vi "Feature Extractor.vi"() -> ()   [LabVIEW 2020]
uses:
  <vilib>/Utility/file.llb/Write Delimited Spreadsheet (string).vi
  <vilib>/Utility/file.llb/Read Delimited Spreadsheet (string).vi
panel:
  in  "Tab Control":enum32{"Measurements", "Settings"}(tab)
  in  "Feature checkmarks":cluster{"Boolean":bool, "String":string}[](array[cluster])=[{"Boolean"=FALSE, "String"="monkey (other animal)"}, {"Boolean"=FALSE, "String"="face (non-face)"}, {"Boolean"=FALSE, "String"="baby (adult)"}]
  in  "next":bool
  in  "previous":bool
  in  "Picture":i32
  out "number of pictures":i32=5
  in  "add object":bool
  in  "save all":bool
  in  "delete object":bool
  in  "next object":bool
  in  "previous object":bool
  in  "Object":i32
  in  "Category":u16(ring) items=["grooming", "aggression", "monkey_play", "group", "mating", "baby_monkey", "animals_playing", "hiding"]
  in  "Save Settings":bool
  in  "Pictures folder path":path=path "C:/Users/Azat/Documents/Monkey Research/Face Grabber/Example"
  in  "Features file path":path=path "C:/Users/Azat/Documents/Monkey Research/Face Grabber/Example/metrics.csv"
  in  "Categories file path":path=path "C:/Users/Azat/Documents/Monkey Research/Face Grabber/Example/stimuli categories.csv"
  in  "show in folder":bool
  in  "new table":bool
  in  "open table":bool
  out "Categories":string[](array[string])=["grooming", "aggression", "monkey_play", "group", "mating", "baby_monkey", "animals_playing", "hiding"]
  out "All Files in Dir":path[](array[path])=[path "C:/Users/Azat/Documents/Monkey Research/Face Grabber/Example/001_monkey_grooming.jpg", path "C:/Users/Azat/Documents/Monkey Research/Face Grabber/Example/017_monkey_aggression.jpg", path "C:/Users/Azat/Documents/Monkey Research/Face Grabber/Example/033_monkey_playing.jpg", path "C:/Users/Azat/Documents/Monkey Research/Face Grabber/Example/049_monkey_group.jpg", path "C:/Users/Azat/Documents/Monkey Research/Face Grabber/Example/089_baby_monkey.jpg"]
  out "Results table":string[][](table)
  in  "Results table file path":path=path "C:/Users/Azat/Documents/Monkey Research/Face Grabber/Example/results.csv"
  out "contours":T1(array[cluster])
  in  "stop":bool
  out "Image":T2(plugin-control)
  # "/"
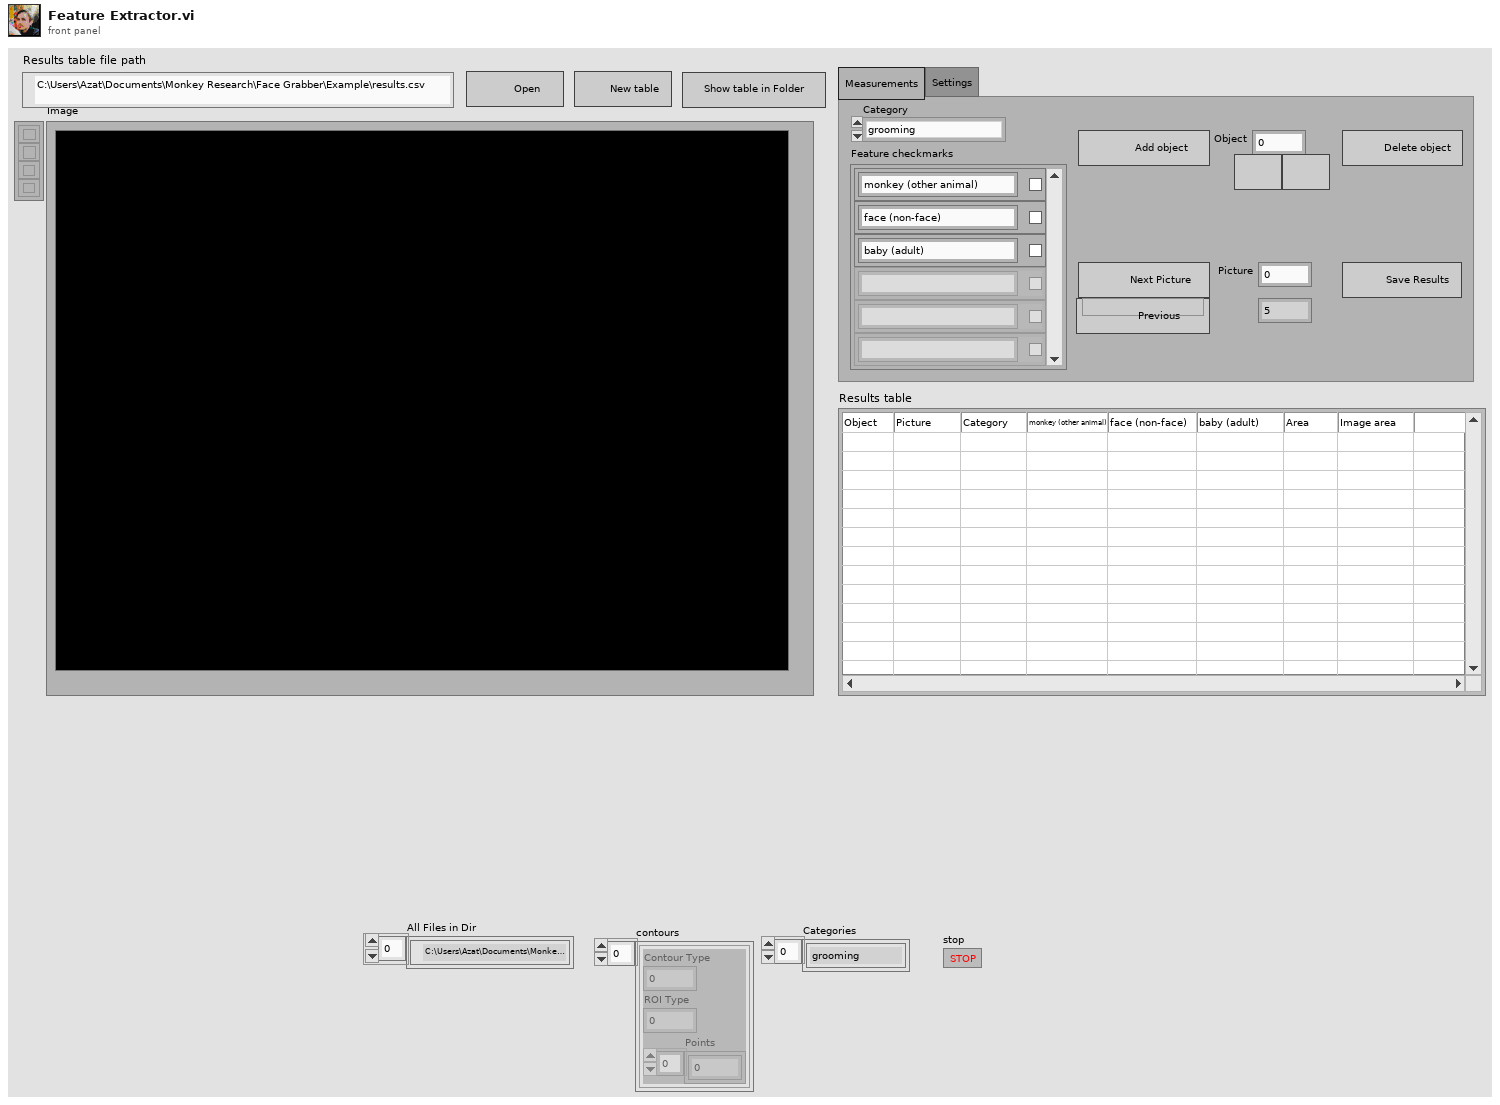
[diagram p1: front panel]
types:
  T1 = cluster{"Contour Type":u32, "ROI Type":u32, "Points":i32[]}[]
  T2 = typedef "IMAQ Image.ctl" = refnum<image>
  T3 = cluster{"Global Rectangle":i32[], "Contours":cluster{"Contour Type":u32, "ROI Type":u32, "Points":i32[]}[]}
  T4 = cluster{"Pictures":path, "results table":path, "Metrics":path, "Categories":path}
  T5 = cluster{"appended path":path, "appended path":path, "appended path":path, "appended path":path}
  T6 = cluster{"[0]":path, "[1]":path, "[2]":path, "[3]":path, "[4]":path, "[5]":path, "[6]":path, "[7]":path, "[8]":path}
  T7 = cluster{"Global Rectangle":i32[], cluster{"Contour Type":u32, "ROI Type":u32, "Points":i32[]}[]}
  T8 = cluster{"Contour Type":u32, "ROI Type":u32, "Points":i32[]}
  T9 = cluster{"Pictures folder path":path, "selected path":path, "Features file path":path, "Categories file path":path}
  T10 = cluster{"Pictures folder path":path, "Results table file path":path, "Features file path":path, "Categories file path":path}
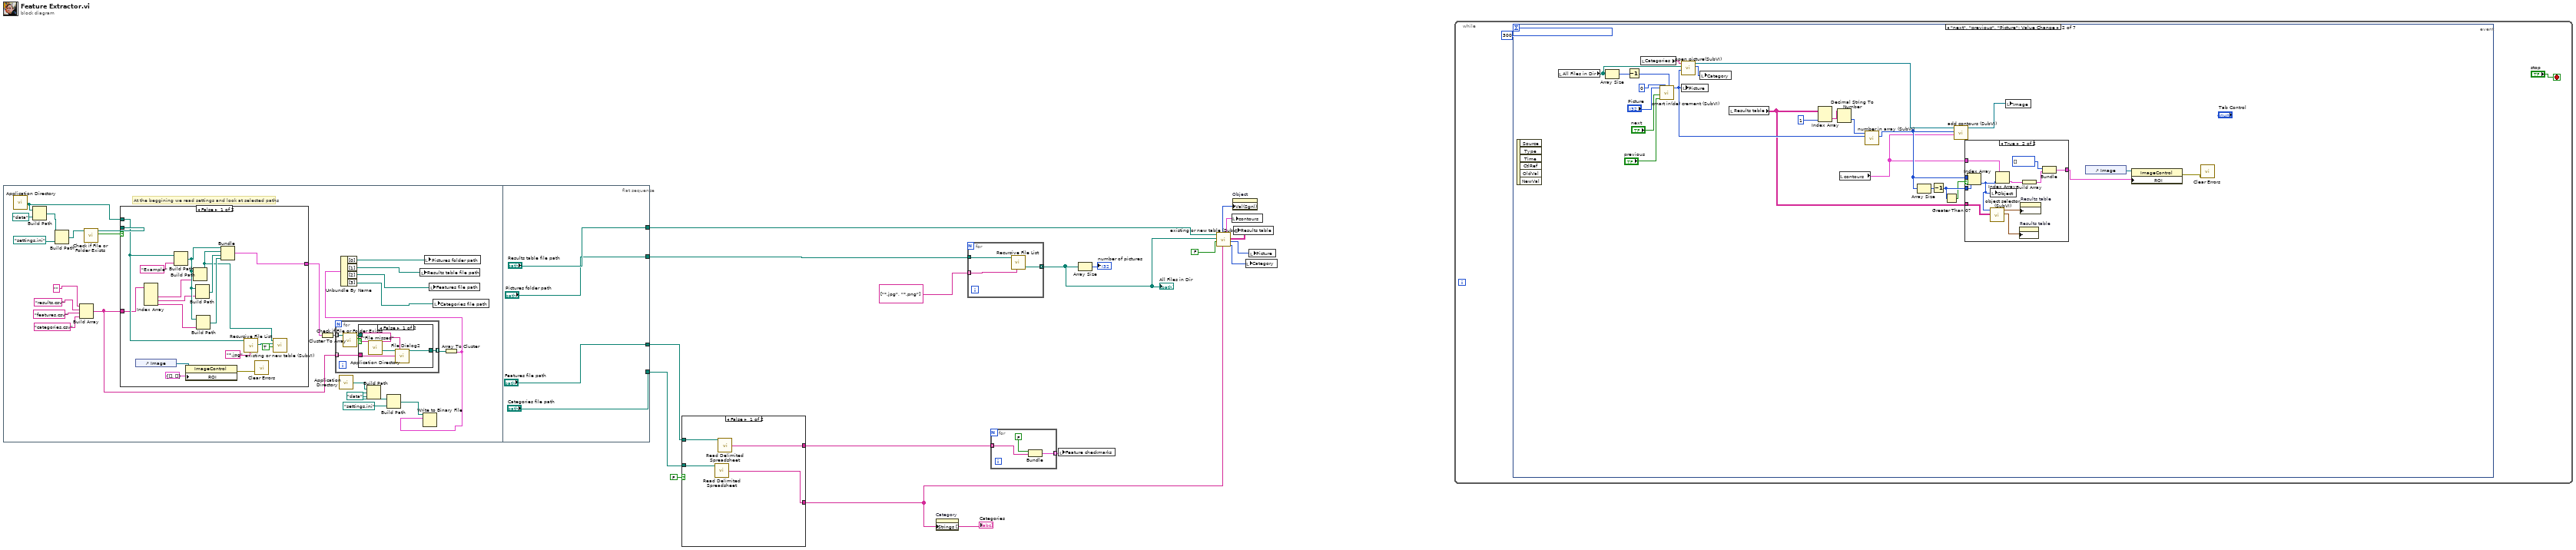
[diagram p0: block diagram]
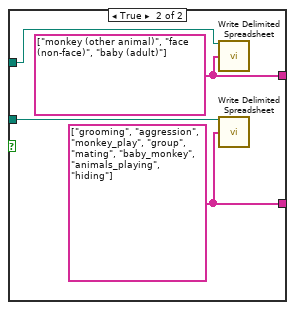
[diagram p2: hidden frame]
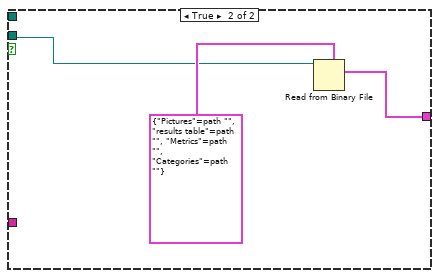
[diagram p4: hidden frame]
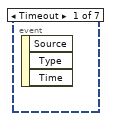
[diagram p5: hidden frame]
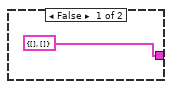
[diagram p6: hidden frame]
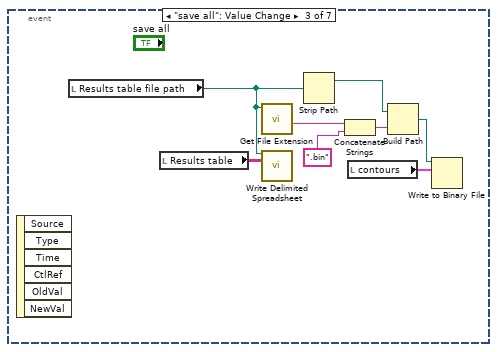
[diagram p7: hidden frame]
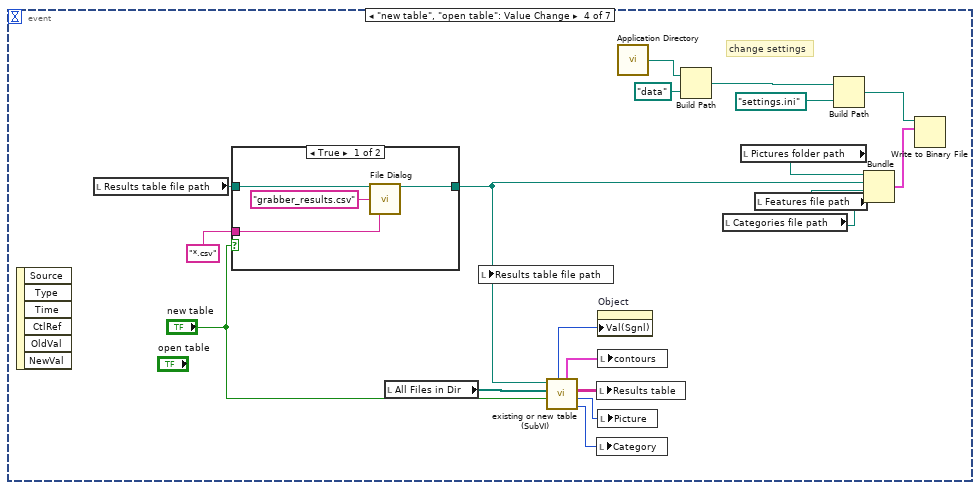
[diagram p8: hidden frame]
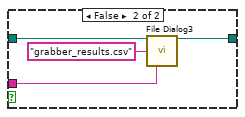
[diagram p9: hidden frame]
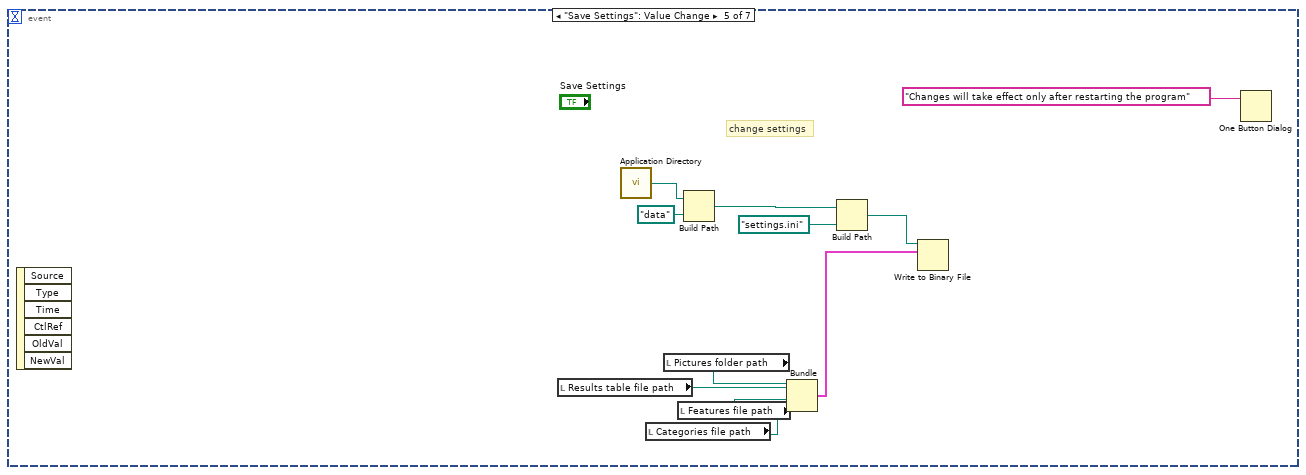
[diagram p10: hidden frame]
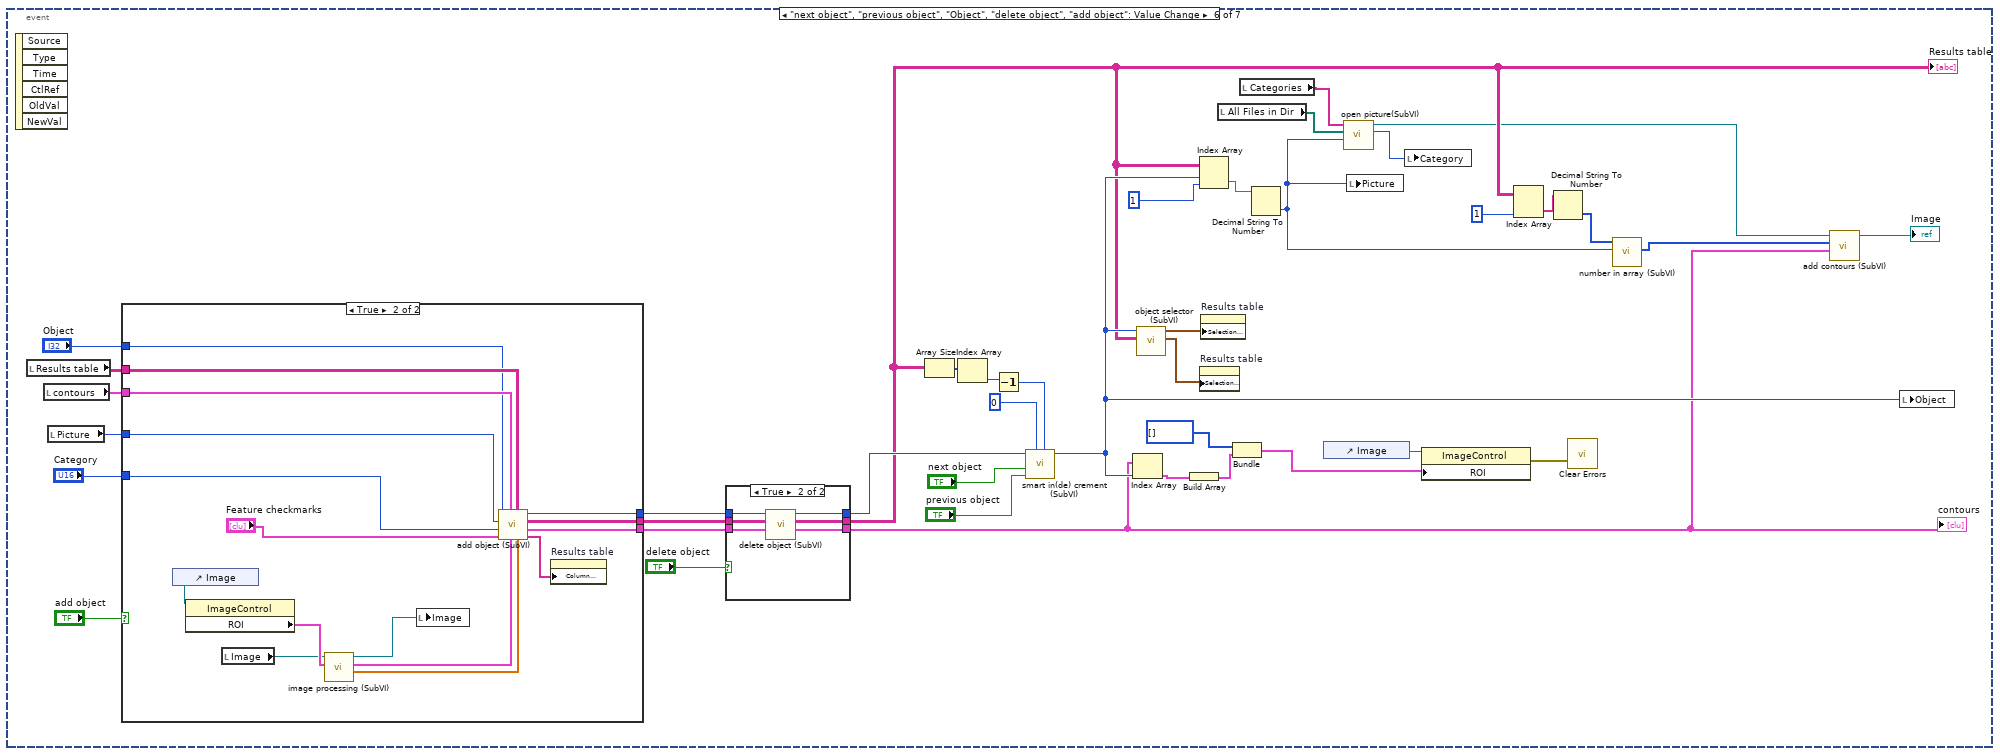
[diagram p11: hidden frame]
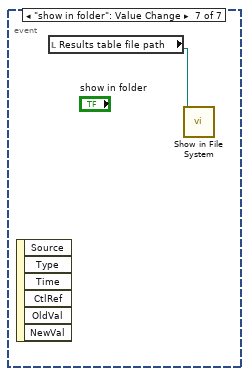
[diagram p14: hidden frame]
diagram:
  n1 = flat-sequence {
    tunnel: ["Results table file path"] -> w11
    tunnel: ["Pictures folder path"] -> w10
    tunnel: ["Features file path"] -> w3
    tunnel: ["Categories file path"] -> w2
    frame #0 {
      # "At the beggining we read settings and look at selected paths"
      n2 = call <vilib>:"Application Directory.vi"() -> ("Application Directory"=w32:path)
      n3 = Build Path(base path=w32, name or relative path=path "data") -> (appended path=w35:path)
      n4 = Build Path(base path=w35, name or relative path=path "settings.ini") -> (appended path=w38:path)
      n5 = Build Array("" ("default name"), "results.csv" ("default name"), "features.csv" ("default name"), "categories.csv" ("default name")) -> (w25:string[])
      n6 = call <vilib>:"Check if File or Folder Exists.vi"("path"=w38) -> ("file or folder exists?"=w39:bool, "dup path"=w40:path)  [unwired: 8 in, 1 out]
      n7 = case shown="False" w39 {
        tunnel: w40 -> [_ w71]
        tunnel: w32 -> [w62 _]
        tunnel: [w69 w70] -> w31
        tunnel: w25 -> [w56 _]
        frame False {
          n8 = control-ref of="Image"() -> (w58:refnum<vi>)
          n9 = Index Array(array=w56) -> (element #2=w55:string, element #3=w54:string, element #4=w53:string)  [unwired: 4 in, 1 out]
          n10 = Build Path(base path=w62, name or relative path="Example" ("default name")) -> (appended path=w65:path)
          n11 = property class="ImageControl"(reference=w58, "ROI"=T3 {"Global Rectangle"=[], "Contours"=[]}) -> (error out=w59:errorcluster)  [unwired: 1 in, 1 out]
          n12 = Build Path(base path=w65, name or relative path=w55) -> (appended path=w60:path)
          n13 = Build Path(base path=w65, name or relative path=w54) -> (appended path=w67:path)
          n14 = Build Path(base path=w65, name or relative path=w53) -> (appended path=w66:path)
          n15 = Bundle("appended path"=w65, "appended path"=w60, "appended path"=w67, "appended path"=w66) -> (w69:T5)  [unwired: 1 in]
          n16 = call <vilib>:"Recursive File List.vi"("pattern"="*.jpg", "Folder Path"=w62) -> ("All Files in Dir"=w63:path[])  [unwired: 5 in, 4 out]
          n17 = call <vilib>:"Clear Errors.vi"("error in (no error)"=w59) -> ()  [unwired: 5 in, 2 out]
          n18 = call "existing or new table (SubVI).vi"("new table?"=TRUE, "All Files in Dir (in)"=w63, "table"=w60) -> ()  [unwired: 4 in, 5 out]
        }
        frame True {
          n19 = Read from Binary File(5:T4 {"Pictures"=path "", "results table"=path "", "Metrics"=path "", "Categories"=path ""} ("output cluster"), 11:w71) -> (2:w70:T4)  [unwired: 4 in, 3 out]
        }
      }
      n20 = Cluster To Array(cluster=w31) -> (array=w30:path[])
      n21 = for {
        tunnel: w30 -> [w47] mode=indexing
        tunnel: w25 -> [w45] mode=indexing
        tunnel: [w43] -> w24 mode=indexing
        n22 = call <vilib>:"Check if File or Folder Exists.vi"("path"=w47) -> ("file or folder exists?"=w46:bool, "dup path"=w44:path)  [unwired: 8 in, 1 out]
        n23 = case shown="False" w46 {
          tunnel: w45 -> [w51 _]
          tunnel: [w48 w52] -> w43
          tunnel: w44 -> [_ w52]
          frame False {
            n24 = call <vilib>:"Application Directory.vi"() -> ("Application Directory"=w49:path)
            n25 = call "File Dialog2"("start path"=w49, "prompt"="File missed", "default name"=w51) -> ("selected path"=w48:path)  [unwired: 9 in, 3 out]
          }
          frame True {
          }
        }
      }
      n26 = call <vilib>:"Application Directory.vi"() -> ("Application Directory"=w22:path)
      n27 = Build Path(base path=w22, name or relative path=path "data") -> (appended path=w21:path)
      n28 = Build Path(base path=w21, name or relative path=path "settings.ini") -> (appended path=w23:path)
      n29 = Array To Cluster(array=w24) -> (cluster=w18:T6)
      n30 = Unbundle By Name(w18) -> ("[0]"=w41:path, "[1]"=w42:path, "[2]"=w34:path, "[3]"=w33:path)
      n31 = local write "Results table file path"(w42) -> ()
      n32 = Write to Binary File(file (use dialog)=w23, data=w18) -> ()  [unwired: 4 in, 3 out]
      n33 = local write "Pictures folder path"(w41) -> ()
      n34 = local write "Features file path"(w34) -> ()
      n35 = local write "Categories file path"(w33) -> ()
    }
    frame #1 {
    }
  }
  n36 = case shown="False" FALSE {
    tunnel: [w77 w81] -> w9
    tunnel: [w79 w84] -> w7
    tunnel: w2 -> [w80 w83]
    tunnel: w3 -> [w78 w82]
    frame False {
      n37 = call-poly <vilib>:"Read Delimited Spreadsheet.vi"("file path (dialog if empty)"=w80) -> ("first row"=w79:string[])  [unwired: 9 in, 5 out]
      n38 = call-poly <vilib>:"Read Delimited Spreadsheet.vi"("file path (dialog if empty)"=w78) -> ("first row"=w77:string[])  [unwired: 9 in, 5 out]
    }
    frame True {
      w81 = string[] ["monkey (other animal)", "face (non-face)", "baby (adult)"]
      w84 = string[] ["grooming", "aggression", "monkey_play", "group", "mating", "baby_monkey", "animals_playing", "hiding"] ("Strings []")
      n39 = call-poly <vilib>:"Write Delimited Spreadsheet.vi"("file path (dialog if empty)"=w82, "1D data"=w81) -> ()  [unwired: 12 in, 2 out]
      n40 = call-poly <vilib>:"Write Delimited Spreadsheet.vi"("file path (dialog if empty)"=w83, "1D data"=w84) -> ()  [unwired: 12 in, 2 out]
    }
  }
  "Categories" <- w7
  n41 = property on="Category" class="Ring (strict)"("Strings []"=w7) -> ()  [unwired: 2 in, 2 out]
  n42 = for {
    tunnel: [w87] -> w12 mode=concatenating
    tunnel: w10 -> [w86]
    tunnel: string[] ["*.jpg", "*.png"] -> [w85] mode=indexing
    n43 = call <vilib>:"Recursive File List.vi"("pattern"=w85, "Folder Path"=w86) -> ("All Files in Dir"=w87:path[])  [unwired: 5 in, 4 out]
  }
  "All Files in Dir" <- w12
  n44 = for {
    tunnel: w9 -> [w89] mode=indexing
    tunnel: [w88] -> w8 mode=indexing
    n45 = Bundle(FALSE, "String"=w89) -> (w88:cluster{bool, "String":string})  [unwired: 1 in]
  }
  n46 = local write "Feature checkmarks"(w8) -> ()
  n47 = Array Size(array=w12) -> (size(s)=→"number of pictures":i32)
  n48 = call "existing or new table (SubVI).vi"("Categories (in)"=w7, "new table?"=FALSE, "All Files in Dir (in)"=w12, "table"=w11) -> ("category"=w13:i32, "picture"=w5:i32, "text table"=w14:string[][], "contours"=w15:T1, "Object"=w4:i32)  [unwired: 3 in]
  n49 = local write "contours"(w15) -> ()
  n50 = property on="Object" class="DigNum (strict)"("Val(Sgnl)"=w4) -> ()  [unwired: 2 in, 2 out]
  n51 = local write "Results table"(w14) -> ()
  n52 = local write "Category"(w13) -> ()
  n53 = local write "Picture"(w5) -> ()
  n54 = while {
    stop <- "stop" stop-if-true
    n55 = event shown="[1] \"next\", \"previous\", \"Picture\": Value Change" {
      selector: _ -> [_ _ _ _ _ _ _]
      dyn-events: _ -> [_ _ _ _ _ _ _]
      timeout: 300 -> [_ _ _ _ _ _ _]
      event Timeout {
        n56 = event-data() -> ()  [unwired: 1 in, 3 out]
      }
      event "next", "previous", "Picture": Value Change {
        n57 = event-data() -> ()  [unwired: 1 in, 6 out]
        n58 = local read "All Files in Dir"() -> (w113:path[])
        n59 = Array Size(array=w113) -> (size(s)=w114:i32)
        n60 = Decrement(x=w114) -> (x-1=w110:i32)
        n61 = local read "Categories"() -> (w115:string[])
        n62 = call "smart in(de) crement (SubVI).vi"("upper limit in"=w110, "lower limit"=0, "previous object"="previous", "next object"="next", "Object"="Picture") -> ("Object out"=w104:i32)  [unwired: 6 in]
        n63 = call "open picture(SubVI).vi"("Picture number"=w104, "All Files in Dir"=w113, "Categories"=w115) -> ("Category"=w116:i32, "Image"=w102:T2)  [unwired: 7 in]
        n64 = local write "Picture"(w104) -> ()
        n65 = local write "Category"(w116) -> ()
        n66 = local read "Results table"() -> (w93:string[][])
        n67 = Index Array(array=w93, index (col)=1 ("disabled index (col)")) -> (element=w106:string[])  [unwired: 1 in]
        n68 = Decimal String To Number(string=w106) -> (number=w105:i32[])  [unwired: 2 in, 1 out]
        n69 = local read "contours"() -> (w99:T1)
        n70 = call "number in array (SubVI).vi"("Numeric"=w104, "Array"=w105) -> ("indexes"=w101:i32[])  [unwired: 8 in, 1 out]
        n71 = Array Size(array=w101) -> (size(s)=w100:i32)
        n72 = Decrement(x=w100) -> (x-1=w98:i32)
        n73 = Greater Than 0?(x=w98) -> (x > 0?=w94:bool)
        n74 = call "add contours (SubVI).vi"("contours in"=w99, "indexes"=w101, "Refnum in"=w102) -> ("Refnum out"=w103:T2)  [unwired: 8 in]
        n75 = case shown="True" w94 {
          tunnel: w101 -> [_ w128]
          tunnel: w99 -> [_ w127]
          tunnel: w98 -> [_ w119]
          tunnel: [T7 {"Global Rectangle"=[], []} ("output cluster") w126] -> w96
          tunnel: w93 -> [_ w120]
          frame False {
          }
          frame True {
            n76 = Index Array(array=w128, index=w119) -> (element=w118:i32)
            n77 = call "object selector (SubVI).vi"("output array"=w120, "Numeric"=w118) -> ("Cluster"=w122:cluster{"Object":i32, i32}, "Cluster 2"=w121:cluster{i32, "Object":i32})  [unwired: 8 in]
            n78 = local write "Object"(w118) -> ()
            n79 = Index Array(array=w127, index=w118) -> (element=w124:T8)
            n80 = property on="Results table" class="Tbl (strict)"("Selection Size"=w122) -> ()  [unwired: 2 in, 2 out]
            n81 = property on="Results table" class="Tbl (strict)"("Selection Start"=w121) -> ()  [unwired: 2 in, 2 out]
            n82 = Build Array(w124) -> (w125:T1)
            n83 = Bundle("Global Rectangle"=i32[] [], w125) -> (w126:T7)  [unwired: 1 in]
          }
        }
        n84 = local write "Image"(w103) -> ()
        n85 = control-ref of="Image"() -> (w95:refnum<vi>)
        n86 = property class="ImageControl"(reference=w95, "ROI"=w96) -> (error out=w97:errorcluster)  [unwired: 1 in, 1 out]
        n87 = call <vilib>:"Clear Errors.vi"("error in (no error)"=w97) -> ()  [unwired: 5 in, 2 out]
      }
      event "save all": Value Change {
        n88 = event-data() -> ()  [unwired: 1 in, 6 out]
        n89 = local read "Results table file path"() -> (w129:path)
        n90 = local read "Results table"() -> (w130:string[][])
        n91 = call <vilib>:"Get File Extension.vi"("file"=w129) -> ("filename without extension"=w135:string)  [unwired: 6 in, 4 out]
        n92 = call-poly <vilib>:"Write Delimited Spreadsheet.vi"("file path (dialog if empty)"=w129, "2D data"=w130) -> ()  [unwired: 12 in, 2 out]
        n93 = Strip Path(path=w129) -> (stripped path=w132:path)  [unwired: 1 out]
        n94 = Concatenate Strings(w135, ".bin" ("string")) -> (w133:string)
        n95 = local read "contours"() -> (w136:T1)
        n96 = Build Path(base path=w132, name or relative path=w133) -> (appended path=w131:path)
        n97 = Write to Binary File(file (use dialog)=w131, data=w136) -> ()  [unwired: 4 in, 3 out]
      }
      event "new table", "open table": Value Change {
        # "change settings"
        n98 = event-data() -> ()  [unwired: 1 in, 6 out]
        n99 = local read "Results table file path"() -> (w148:path)
        n100 = case shown="True" "new table" {
          tunnel: [w159 w163] -> w143
          tunnel: w148 -> [w157 w161]
          tunnel: "*.csv" ("pattern (all files)") -> [w156 w160]
          frame True {
            n101 = call "File Dialog"("start path"=w157, "default name"="grabber_results.csv", "pattern (all files)"=w156) -> ("selected path"=w159:path)  [unwired: 9 in, 3 out]
          }
          frame False {
            n102 = call "File Dialog3"("start path"=w161, "default name"="grabber_results.csv", "pattern (all files)"=w160) -> ("selected path"=w163:path)  [unwired: 9 in, 3 out]
          }
        }
        n103 = local read "All Files in Dir"() -> (w149:path[])
        n104 = local write "Results table file path"(w143) -> ()
        n105 = call "existing or new table (SubVI).vi"("new table?"="new table", "All Files in Dir (in)"=w149, "table"=w143) -> ("category"=w150:i32, "picture"=w151:i32, "text table"=w152:string[][], "contours"=w146:T1, "Object"=w142:i32)  [unwired: 4 in]
        n106 = local write "Results table"(w152) -> ()
        n107 = local write "Category"(w150) -> ()
        n108 = property on="Object" class="DigNum (strict)"("Val(Sgnl)"=w142) -> ()  [unwired: 2 in, 2 out]
        n109 = local write "contours"(w146) -> ()
        n110 = local write "Picture"(w151) -> ()
        n111 = call <vilib>:"Application Directory.vi"() -> ("Application Directory"=w138:path)
        n112 = Build Path(base path=w138, name or relative path=path "data") -> (appended path=w137:path)
        n113 = local read "Categories file path"() -> (w140:path)
        n114 = local read "Pictures folder path"() -> (w144:path)
        n115 = local read "Features file path"() -> (w141:path)
        n116 = Build Path(base path=w137, name or relative path=path "settings.ini") -> (appended path=w154:path)
        n117 = Bundle("Pictures folder path"=w144, "selected path"=w143, "Features file path"=w141, "Categories file path"=w140) -> (w155:T9)  [unwired: 1 in]
        n118 = Write to Binary File(file (use dialog)=w154, data=w155) -> ()  [unwired: 4 in, 3 out]
      }
      event "Save Settings": Value Change {
        # "change settings"
        n119 = event-data() -> ()  [unwired: 1 in, 6 out]
        n120 = local read "Results table file path"() -> (w165:path)
        n121 = call <vilib>:"Application Directory.vi"() -> ("Application Directory"=w169:path)
        n122 = local read "Categories file path"() -> (w170:path)
        n123 = local read "Pictures folder path"() -> (w172:path)
        n124 = local read "Features file path"() -> (w171:path)
        n125 = Build Path(base path=w169, name or relative path=path "data") -> (appended path=w168:path)
        n126 = Bundle("Pictures folder path"=w172, "Results table file path"=w165, "Features file path"=w171, "Categories file path"=w170) -> (w174:T10)  [unwired: 1 in]
        n127 = Build Path(base path=w168, name or relative path=path "settings.ini") -> (appended path=w173:path)
        n128 = Write to Binary File(file (use dialog)=w173, data=w174) -> ()  [unwired: 4 in, 3 out]
        n129 = One Button Dialog(message="Changes will take effect only after restarting the program") -> ()  [unwired: 1 in, 1 out]
      }
      event "next object", "previous object", "Object", "delete object", "add object": Value Change {
        n130 = event-data() -> ()  [unwired: 1 in, 6 out]
        n131 = local read "Results table"() -> (w196:string[][])
        n132 = local read "contours"() -> (w197:T1)
        n133 = local read "Picture"() -> (w182:i32)
        n134 = case shown="True" "add object" {
          tunnel: [w225 w235] -> w200
          tunnel: [w224 w234] -> w199
          tunnel: [w226 w233] -> w198
          tunnel: w197 -> [w225 w231]
          tunnel: w196 -> [w226 w230]
          tunnel: "Object" -> [w224 w229]
          tunnel: w182 -> [_ w228]
          tunnel: "Category" -> [_ w227]
          frame False {
          }
          frame True {
            n135 = control-ref of="Image"() -> (w232:refnum<vi>)
            n136 = property class="ImageControl"(reference=w232) -> ("ROI"=w241:T3)  [unwired: 1 in, 2 out]
            n137 = local read "Image"() -> (w238:T2)
            n138 = call "image processing (SubVI).vi"("ROI"=w241, "Refnum in"=w238) -> ("Particle Measurements (Pixels)"=w236:dbl[], "Cluster"=w242:T8, "Image Out (duplicate)"=w237:T2)  [unwired: 7 in]
            n139 = local write "Image"(w237) -> ()
            n140 = call "add object (SubVI).vi"("Particle Measurements (Pixels)"=w236, "output array in"=w230, "Cluster"=w242, "contours in"=w231, "metrics"="Feature checkmarks", "category"=w227, "Picture"=w228, "Object in"=w229) -> ("Array"=w239:string[], "contours out"=w235:T1, "output array out"=w233:string[][], "Object out"=w234:i32)
            n141 = property on="Results table" class="Tbl (strict)"("Column Headers[]"=w239) -> ()  [unwired: 2 in, 2 out]
          }
        }
        n142 = case shown="True" "delete object" {
          tunnel: w200 -> [w215 w223]
          tunnel: w199 -> [w217 w222]
          tunnel: w198 -> [w216 w221]
          tunnel: [w216 w220] -> w190
          tunnel: [w215 w219] -> w184
          tunnel: [w217 w218] -> w192
          frame False {
          }
          frame True {
            n143 = call "delete object (SubVI).vi"("contours in"=w223, "output array in"=w221, "Object"=w222) -> ("contours out"=w219:T1, "output array out"=w220:string[][], "Object"=w218:i32)  [unwired: 6 in]
          }
        }
        "contours" <- w184
        "Results table" <- w190
        n144 = Array Size(array=w190) -> (size(s)=w207:i32[])
        n145 = Index Array(array=w207) -> (element=w206:i32)  [unwired: 1 in]
        n146 = Decrement(x=w206) -> (x-1=w201:i32)
        n147 = call "smart in(de) crement (SubVI).vi"("upper limit in"=w201, "lower limit"=0, "previous object"="previous object", "next object"="next object", "Object"=w192) -> ("Object out"=w204:i32)  [unwired: 6 in]
        n148 = Index Array(array=w184, index=w204) -> (element=w178:T8)
        n149 = call "object selector (SubVI).vi"("output array"=w190, "Numeric"=w204) -> ("Cluster"=w203:cluster{"Object":i32, i32}, "Cluster 2"=w202:cluster{i32, "Object":i32})  [unwired: 8 in]
        n150 = Build Array(w178) -> (w177:T1)
        n151 = Index Array(array=w190, index (row)=w204, index (col)=1 ("disabled index (col)")) -> (element=w205:string)
        n152 = property on="Results table" class="Tbl (strict)"("Selection Size"=w203) -> ()  [unwired: 2 in, 2 out]
        n153 = property on="Results table" class="Tbl (strict)"("Selection Start"=w202) -> ()  [unwired: 2 in, 2 out]
        n154 = local read "All Files in Dir"() -> (w191:path[])
        n155 = Bundle("Global Rectangle"=i32[] [], w177) -> (w176:T7)  [unwired: 1 in]
        n156 = local read "Categories"() -> (w210:string[])
        n157 = Decimal String To Number(string=w205) -> (number=w186:i32)  [unwired: 2 in, 1 out]
        n158 = control-ref of="Image"() -> (w209:refnum<vi>)
        n159 = call "open picture(SubVI).vi"("Picture number"=w186, "All Files in Dir"=w191, "Categories"=w210) -> ("Category"=w211:i32, "Image"=w183:T2)  [unwired: 7 in]
        n160 = local write "Picture"(w186) -> ()
        n161 = local write "Category"(w211) -> ()
        n162 = property class="ImageControl"(reference=w209, "ROI"=w176) -> (error out=w175:errorcluster)  [unwired: 1 in, 1 out]
        n163 = Index Array(array=w190, index (col)=1 ("disabled index (col)")) -> (element=w188:string[])  [unwired: 1 in]
        n164 = Decimal String To Number(string=w188) -> (number=w187:i32[])  [unwired: 2 in, 1 out]
        n165 = call <vilib>:"Clear Errors.vi"("error in (no error)"=w175) -> ()  [unwired: 5 in, 2 out]
        n166 = call "number in array (SubVI).vi"("Numeric"=w186, "Array"=w187) -> ("indexes"=w185:i32[])  [unwired: 8 in, 1 out]
        n167 = call "add contours (SubVI).vi"("contours in"=w184, "indexes"=w185, "Refnum in"=w183) -> ("Refnum out"=→"Image":T2)  [unwired: 8 in]
        n168 = local write "Object"(w204) -> ()
      }
      event "show in folder": Value Change {
        n169 = event-data() -> ()  [unwired: 1 in, 6 out]
        n170 = local read "Results table file path"() -> (w243:path)
        n171 = call <vilib>:"Show in File System.vi"("file or directory path"=w243) -> ()  [unwired: 10 in, 1 out]
      }
    }
  }
